vi "Running Average.vi"(9 "Points Averaged":dbl, 10 "Running average":dbl, 11 "notification":dbl[](array[numeric])) -> (2 "Points Avged Out":dbl, 3 "Running Avg Out":dbl)   [LabVIEW 2013, in "Feedback.lvlib"]
uses:
  Feedback.lvlib
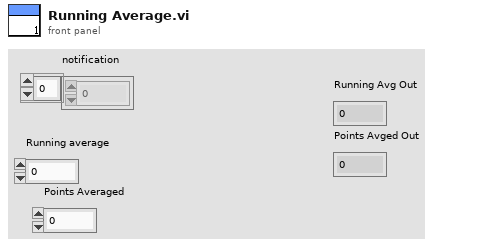
[diagram p1: front panel]
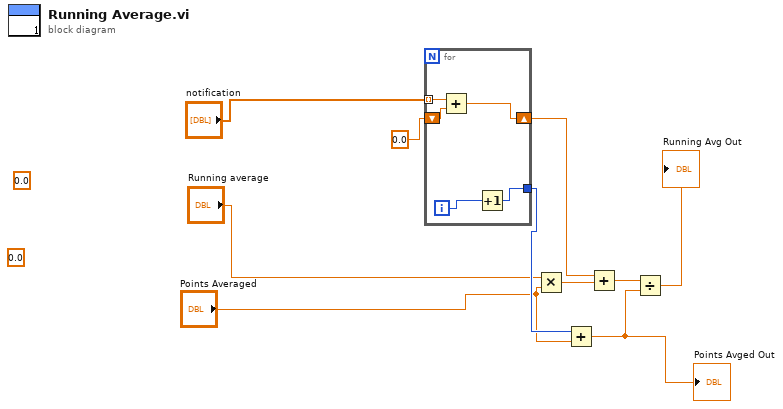
[diagram p0: block diagram]
diagram:
  (unwired) 0.0 ("Avging window")
  (unwired) 0.0 ("Last Update Time")
  n1 = for {
    tunnel: "notification" -> [w15] mode=indexing
    shift-right: [w13] -> w8
    shift-left: 0.0 ("y") -> [w14]
    tunnel: [w11] -> w6
    i -> [w12]
    n2 = Add(x=w15, y=w14) -> (x+y=w13:dbl)
    n3 = Increment(x=w12) -> (x+1=w11:i32)
  }
  n4 = Multiply(x="Running average", y="Points Averaged") -> (x*y=w9:dbl)
  n5 = Add(x=w6, y="Points Averaged") -> (x+y=w4:dbl)
  "Points Avged Out" <- w4
  n6 = Add(x=w8, y=w9) -> (x+y=w7:dbl)
  n7 = Divide(x=w7, y=w4) -> (x/y=→"Running Avg Out":dbl)
